vi "Quick Usb Write Data Async.vi"(7 "transaction":string, 8 "error in (no error)":errorcluster, 9 "length":u32, 10 "data":string, 11 "hDevice":u32) -> (0 "error out":errorcluster, 1 "function return":i32, 2 "data out":string, 3 "hDevice out":u32, 5 "transaction out":string)   [LabVIEW 2011, in "QuickUSB.lvlib"]
doc: "QUSBLIB QRETURN QuickUsbWriteDataAsync(\n QHANDLE hDevice, \n PQBYTE data, \n QULONG length, \n PQBYTE transaction\n);"
uses:
  QuickUSB.lvlib
  QuickUSB.dll
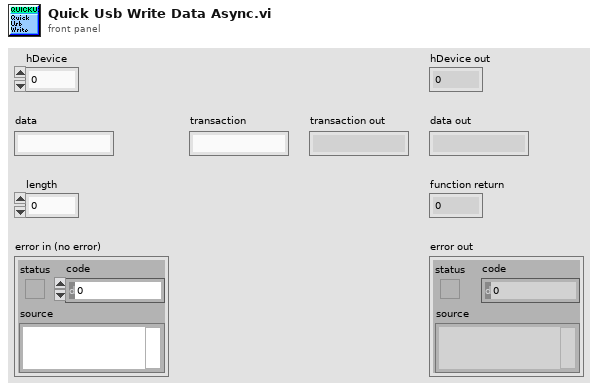
[diagram p1: front panel]
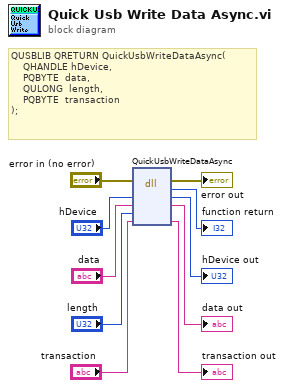
[diagram p0: block diagram]
diagram:
  # "QUSBLIB QRETURN QuickUsbWriteDataAsync(\n    QHANDLE hDevice, \n    PQBYTE  data, \n    QULONG  length, \n    PQBYTE  transaction\n);"
  n1 = dll-call lib="C:/QuickUSB/QuickUSB.*" fn="QuickUsbWriteDataAsync"(error in="error in (no error)", "hDevice"="hDevice", "data"="data", "length"="length", "transaction"="transaction") -> (error out=→"error out":errorcluster, →"function return":i32, "hDevice"=→"hDevice out":u32, "data"=→"data out":string, "transaction"=→"transaction out":string)  [unwired: 3 in, 1 out]
